vi "Module Init.vi"(8 "error in (no error)":errorcluster, 11 "Remote Messaging Module in":refnum<class "Remote Messaging Module.lvclass">) -> (0 "error out":errorcluster, 3 "Remote Messaging Module out":refnum<class "Remote Messaging Module.lvclass">)   [LabVIEW 2020, in "Volatus.lvlib" / "Remote Messaging Module.lvclass"]
uses:
  Remote Messaging Module.lvclass
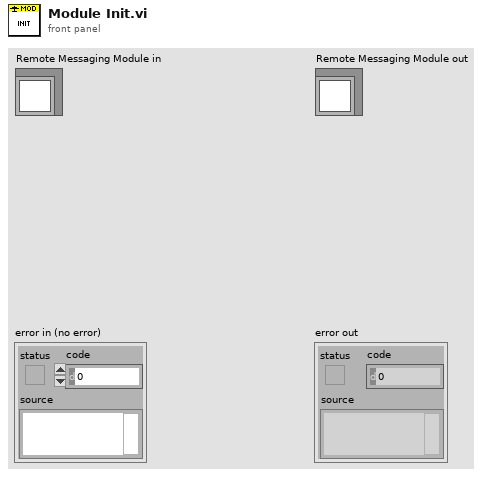
[diagram p1: front panel]
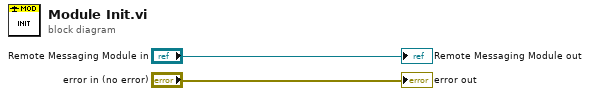
[diagram p0: block diagram]
diagram:
  "error out" <- "error in (no error)"
  "Remote Messaging Module out" <- "Remote Messaging Module in"
